vi "tutorial 1.vi"() -> ()   [LabVIEW 2022 SP3]
panel:
  in  "stop":bool
  out "output":dbl
  in  "input2":dbl
  in  "input1":dbl
  in  "function name":string
  in  "Python path":path
  in  "Python version":string
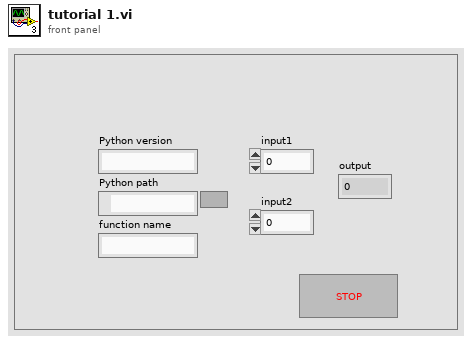
[diagram p1: front panel]
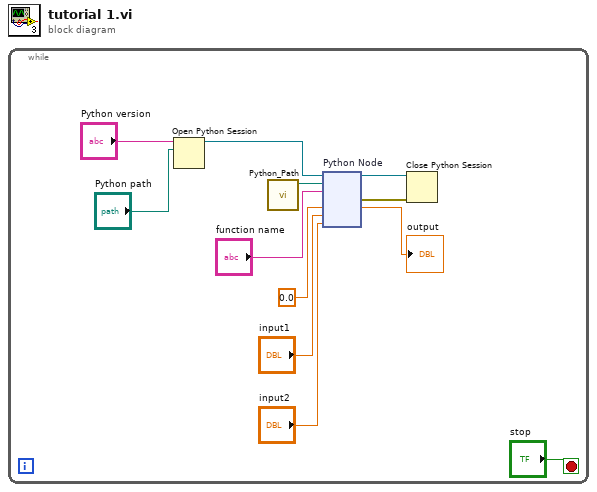
[diagram p0: block diagram]
diagram:
  n1 = while {
    stop <- "stop" stop-if-true
    n2 = Open Python Session(python version="Python version", python path="Python path") -> (session out=w10:refnum<k35>)  [unwired: 1 in, 1 out]
    n3 = call "Python_Path.vi"() -> ("appended path"=w9:path)  [unwired: 11 in]
    n4 = node "Python Node"(w10, w9, "function name", 0.0, "input1", "input2") -> (w4:refnum<k35>, w2:errorcluster, →"output":dbl)  [unwired: 3 in, 2 out]
    n5 = Close Python Session(session in=w4, error in=w2) -> ()  [unwired: 1 out]
  }
